vi "Read INI Section 2.vi"(4 "error IN":errorcluster, 5 "Sort":bool=TRUE, 6 "section":string="Manufacturer", 7 "configuration file path":path) -> (0 "error OUT":errorcluster, 3 "Array":string[](array[string]))   [LabVIEW 2015]
uses:
  <vilib>/Utility/config.llb/Read Key (String).vi
  <vilib>/Utility/config.llb/NI_LVConfig.lvlib
panel:
  # "Sorted"
  # "Unsorted"
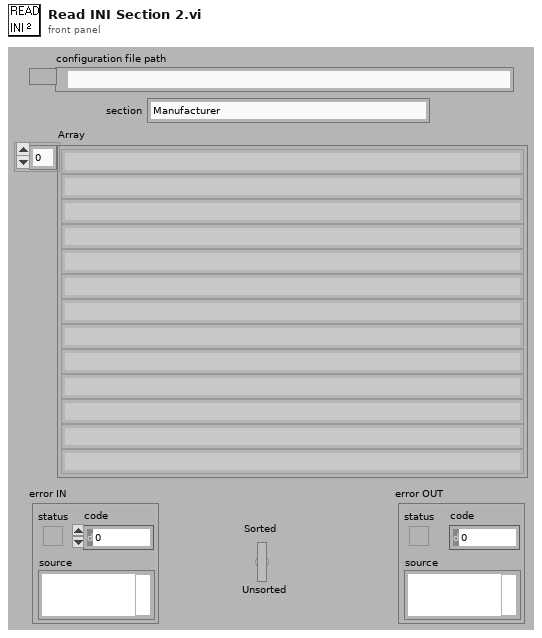
[diagram p1: front panel]
types:
  T1 = typedef "NI_LVConfig.lvlib/Config Data RefNum.ctl" = refnum<k1>
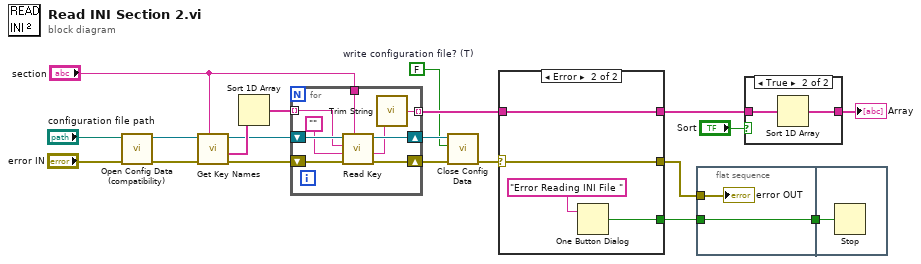
[diagram p0: block diagram]
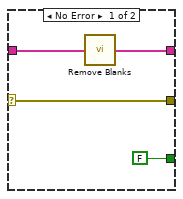
[diagram p3: hidden frame]
diagram:
  w4 = FALSE  # write configuration file? (T)
  n1 = call <vilib>:"Open Config Data (compatibility).vi"("error in (no error)"="error IN", "configuration file path"="configuration file path") -> ("error out"=w13:errorcluster, "refnum"=w14:T1)  [unwired: 7 in, 1 out]
  n2 = call <vilib>:"Get Key Names.vi"("section"="section", "error in (no error)"=w13, "refnum"=w14) -> ("error out"=w18:errorcluster, "key names"=w16:string[], "refnum out"=w15:T1)  [unwired: 6 out]
  n3 = Sort 1D Array(array=w16) -> (sorted array=w5:string[])
  n4 = for {
    tunnel: w5 -> [w27] mode=indexing
    tunnel: "section" -> [w24]
    tunnel: [w21] -> w8 mode=indexing
    shift-right: [w22] -> w12
    shift-left: w18 -> [w26]
    shift-right: [w28] -> w17
    shift-left: w15 -> [w29]
    n5 = call-poly <vilib>:"Read Key.vi"("section"=w24, "error in (no error)"=w26, "default value"="", "key"=w27, "refnum"=w29) -> ("error out"=w22:errorcluster, "value"=w23:string, "refnum out"=w28:T1)  [unwired: 1 in, 3 out]
    n6 = call "Trim String.vi"("inStr"=w23) -> ("outStr"=w21:string)
  }
  n7 = call <vilib>:"Close Config Data.vi"("error in (no error)"=w12, "write file if changed (T)"=w4, "refnum"=w17) -> ("error out"=w11:errorcluster)  [unwired: 8 out]
  n8 = case shown="Error" w11 {
    selector: w11 -> [w31 w35]
    tunnel: w8 -> [w33 w36]
    tunnel: [w32 w36] -> w6
    tunnel: [w31 w35] -> w2
    tunnel: [FALSE ("true") w34] -> w3
    frame No Error {
      n9 = call "Remove Blanks.vi"("INPUT STRING ARRAY"=w33) -> ("OUTPUT STRING ARRAY"=w32:string[])
    }
    frame Error {
      n10 = One Button Dialog(message="Error Reading INI File ") -> (true=w34:bool)  [unwired: 1 out]
    }
  }
  n11 = flat-sequence {
    tunnel: w3 -> [w39]
    tunnel: w2 -> [w38]
    tunnel: [w39] -> w1
    tunnel: w1 -> [w40]
    frame #0 {
      "error OUT" <- w38
    }
    frame #1 {
      n12 = Stop(stop? (T)=w40) -> ()
    }
  }
  n13 = case shown="True" "Sort" {
    tunnel: w6 -> [w41 w43]
    tunnel: [w41 w42] -> w9
    frame False {
    }
    frame True {
      n14 = Sort 1D Array(array=w43) -> (sorted array=w42:string[])
    }
  }
  "Array" <- w9
